vi "Simulator.vi"(8 "Run button":bool, 10 "Reads":u8[](array[numeric]), 11 "Commands":u8[](array[numeric])) -> (3 "Writes":u8[](array[numeric]))   [LabVIEW 2018]
uses:
  <vilib>/rvi/interface/RandomDataEmulation/nirviRandomDataOpen.vi
  <vilib>/rvi/interface/common/niFpgaCacheSessionInfoDynamic.vi
  <vilib>/FPGAPlugInAG/Dynamic/niLvFpga_Run_Dynamic.vi
  <vilib>/Utility/error.llb/Error Cluster From Error Code.vi
  <vilib>/rvi/errors/niLvFpgaAdjustHostInterfaceError.vi
  <vilib>/FPGAPlugInAG/Dynamic/niLvFpga_Close_Dynamic.vi
  <vilib>/rvi/interface/nirviOpenFPGA/nirviOpenFPGA.xnode
  FPGATest.vi
  <vilib>/rvi/interface/nirviMethod/nirviMethod.xnode
  <vilib>/rvi/interface/nirviCloseFPGA/nirviCloseFPGA.xnode
  <vilib>/FPGAPlugInAG/Dynamic/niLvFpga_WriteFifo_Dynamic.vi
  <vilib>/rvi/errors/niLvFpgaMergeErrorWithErrorCode.vi
  <vilib>/FPGAPlugInAG/Dynamic/niLvFpga_ReadFifo_Dynamic.vi
panel:
  out "Readouts":u8[](array[numeric])
  in  "stop":bool
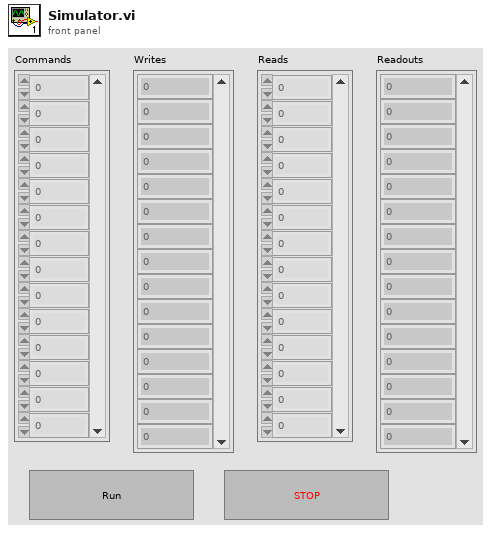
[diagram p1: front panel]
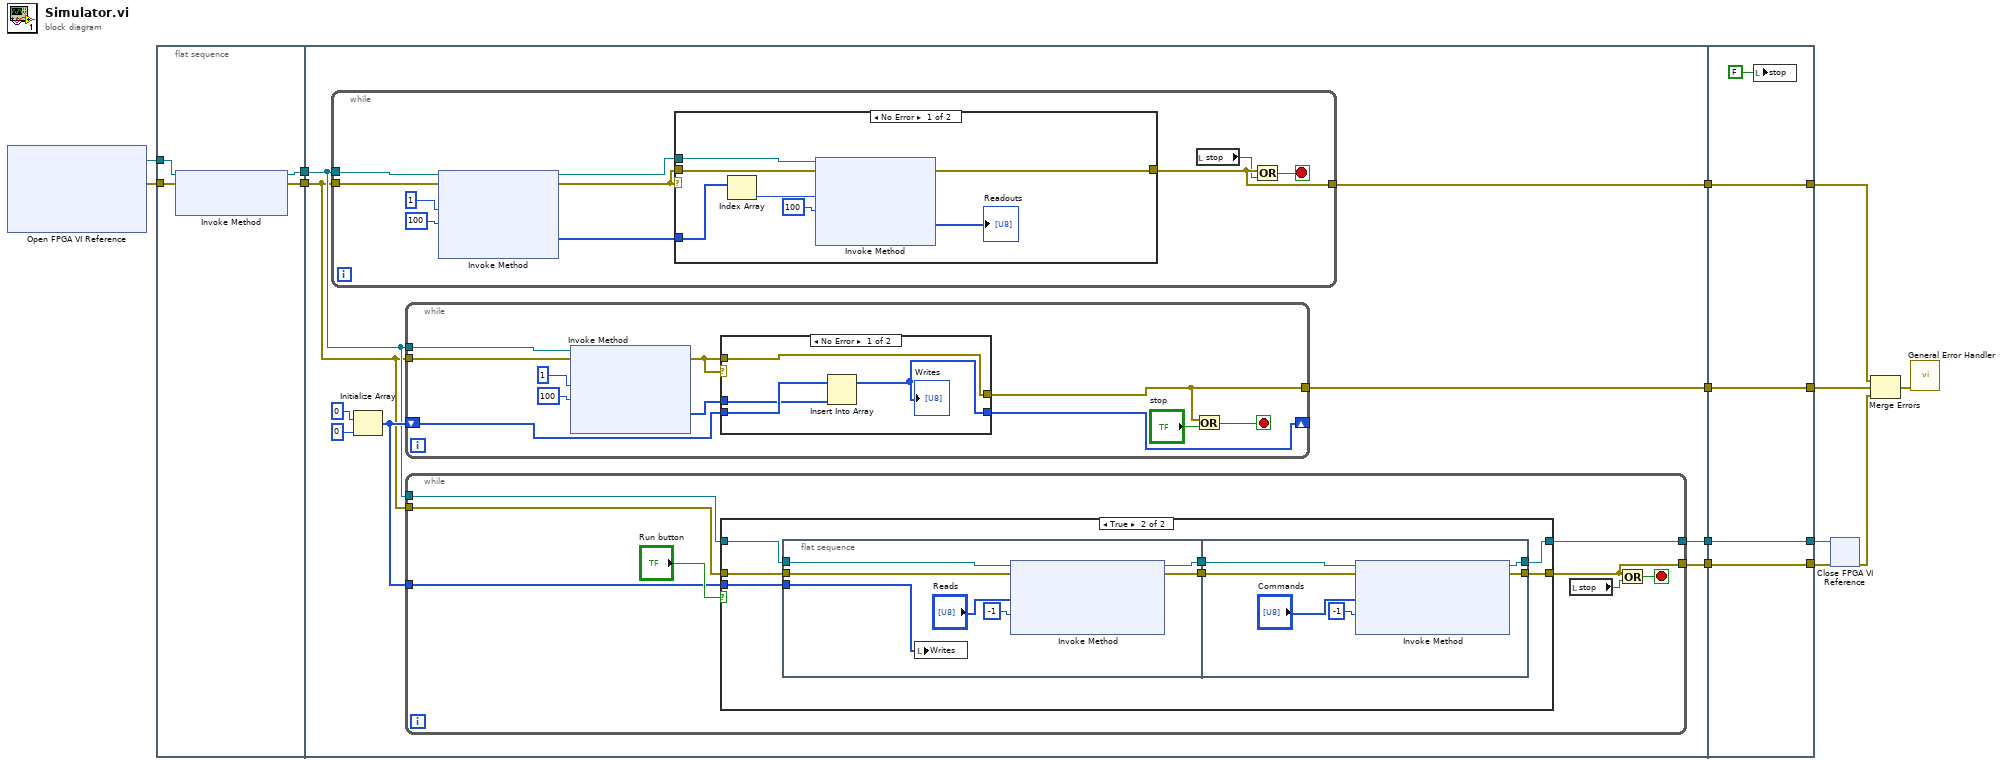
[diagram p0: block diagram]
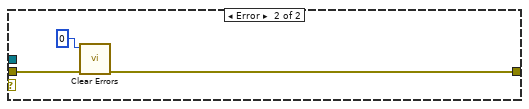
[diagram p2: hidden frame]
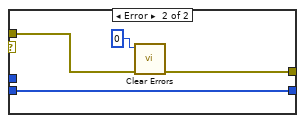
[diagram p3: hidden frame]
diagram:
  n1 = xnode "Open FPGA VI Reference"() -> ("FPGA VI Reference Out"=w14:refnum<k20>, "error out"=w13:errorcluster)  [unwired: 2 in]
  n2 = flat-sequence {
    tunnel: w13 -> [w17]
    tunnel: w14 -> [w18]
    tunnel: [w16] -> w10
    tunnel: [w15] -> w9
    tunnel: w10 -> [w20]
    tunnel: w9 -> [w21]
    tunnel: [w27] -> w5
    tunnel: [w26] -> w4
    tunnel: [w23] -> w3
    tunnel: [w19] -> w2
    tunnel: [w99] -> w6
    tunnel: [w100] -> w11
    tunnel: [w101] -> w12
    tunnel: w5 -> [w101]
    tunnel: w4 -> [w100]
    tunnel: w3 -> [w99]
    tunnel: [w97] -> w1
    tunnel: w2 -> [w97]
    frame #0 {
      n3 = xnode "Invoke Method"("FPGA VI Reference In"=w18, "error in"=w17) -> ("FPGA VI Reference Out"=w15:refnum<k20>, "error out"=w16:errorcluster)  [unwired: 1 in]
    }
    frame #1 {
      n4 = while {
        tunnel: w21 -> [w37]
        tunnel: w20 -> [w36]
        tunnel: [w30] -> w19
        stop <- w32 stop-if-true
        n5 = xnode "Invoke Method"("FPGA VI Reference In"=w37, "error in"=w36, "Number of Elements"=u32 1, "Timeout (ms)"=100) -> ("FPGA VI Reference Out"=w31:refnum<k20>, "error out"=w29:errorcluster, "Data"=w33:u8[])  [unwired: 1 out]
        n6 = case shown="No Error" w29 {
          tunnel: w33 -> [w44 _]
          tunnel: w29 -> [w42 w46]
          tunnel: w31 -> [w41 _]
          tunnel: [w38 w45] -> w30
          frame No Error {
            n7 = Index Array(array=w44) -> (element=w43:u8)  [unwired: 1 in]
            n8 = xnode "Invoke Method"("FPGA VI Reference In"=w41, "error in"=w42, "Number of Elements"=w43, "Timeout (ms)"=100) -> ("error out"=w38:errorcluster, "Data"=→"Readouts":u8[])  [unwired: 2 out]
          }
          frame Error {
            n9 = call <vilib>:"Clear Errors.vi"("error in (no error)"=w46, "specific error code to clear (0: all)"=0) -> ("error out"=w45:errorcluster)  [unwired: 4 in, 1 out]
          }
        }
        n10 = local read "stop"() -> (w28:bool)
        n11 = Or(x=w30, y=w28) -> (x .or. y?=w32:bool)
      }
      n12 = Initialize Array(u8 0 ("element"), 0 ("dimension size")) -> (w22:u8[])
      n13 = while {
        tunnel: w21 -> [w55]
        tunnel: w20 -> [w56]
        tunnel: [w50] -> w23
        shift-right: [w48] -> _
        shift-left: w22 -> [w54]
        stop <- w51 stop-if-true
        n14 = xnode "Invoke Method"("FPGA VI Reference In"=w55, "error in"=w56, "Number of Elements"=u32 1, "Timeout (ms)"=100) -> ("error out"=w49:errorcluster, "Data"=w53:u8[])  [unwired: 2 out]
        n15 = case shown="No Error" w49 {
          tunnel: w54 -> [w62 w66]
          tunnel: w53 -> [w61 _]
          tunnel: [w60 w66] -> w48
          tunnel: [w59 w64] -> w50
          tunnel: w49 -> [w59 w65]
          frame No Error {
            n16 = Insert Into Array(array=w62, new element=w61) -> (w60:u8[])  [unwired: 1 in]
            "Writes" <- w60
          }
          frame Error {
            n17 = call <vilib>:"Clear Errors.vi"("error in (no error)"=w65, "specific error code to clear (0: all)"=0) -> ("error out"=w64:errorcluster)  [unwired: 4 in, 1 out]
          }
        }
        n18 = Or(x=w50, y="stop") -> (x .or. y?=w51:bool)
      }
      n19 = while {
        tunnel: w20 -> [w71]
        tunnel: [w67] -> w26
        tunnel: w21 -> [w72]
        tunnel: [w73] -> w27
        tunnel: w22 -> [w69]
        stop <- w68 stop-if-true
        n20 = case shown="True" "Run button" {
          tunnel: w72 -> [w76 w83]
          tunnel: [w76 w82] -> w73
          tunnel: [w75 w81] -> w67
          tunnel: w71 -> [w75 w80]
          tunnel: w69 -> [_ w78]
          frame False {
          }
          frame True {
            n21 = flat-sequence {
              tunnel: w80 -> [w84]
              tunnel: w83 -> [w90]
              tunnel: [w89] -> w79
              tunnel: w78 -> [w86]
              tunnel: [w85] -> w77
              tunnel: [w95] -> w82
              tunnel: [w94] -> w81
              tunnel: w79 -> [w96]
              tunnel: w77 -> [w93]
              frame #0 {
                n22 = local write "Writes"(w86) -> ()
                n23 = xnode "Invoke Method"("FPGA VI Reference In"=w90, "error in"=w84, "Data"="Reads", "Timeout (ms)"=-1) -> ("FPGA VI Reference Out"=w89:refnum<k20>, "error out"=w85:errorcluster)  [unwired: 1 out]
              }
              frame #1 {
                n24 = xnode "Invoke Method"("FPGA VI Reference In"=w96, "error in"=w93, "Data"="Commands", "Timeout (ms)"=-1) -> ("FPGA VI Reference Out"=w95:refnum<k20>, "error out"=w94:errorcluster)  [unwired: 1 out]
              }
            }
          }
        }
        n25 = local read "stop"() -> (w70:bool)
        n26 = Or(x=w67, y=w70) -> (x .or. y?=w68:bool)
      }
    }
    frame #2 {
      n27 = local write "stop"(FALSE ("stop")) -> ()
    }
  }
  n28 = xnode "Close FPGA VI Reference"("FPGA VI Reference In"=w12, "error in"=w11) -> ("error out"=w7:errorcluster)
  n29 = Merge Errors(w1, w6, w7) -> (w8:errorcluster)
  n30 = call <vilib>:"General Error Handler.vi"("error in (no error)"=w8) -> ()  [unwired: 10 in, 5 out]
